vi "WriteSF.vi"(4 "error in":errorcluster, 5 "packet":u8[](array[numeric]), 6 "Enablle write":bool, 7 "connection ID":refnum<k5>) -> (0 "error out":errorcluster, 1 "Bytes written to SF":dbl, 2 "Packet String":string, 3 "connection ID out":refnum<k5>)   [LabVIEW 2011]
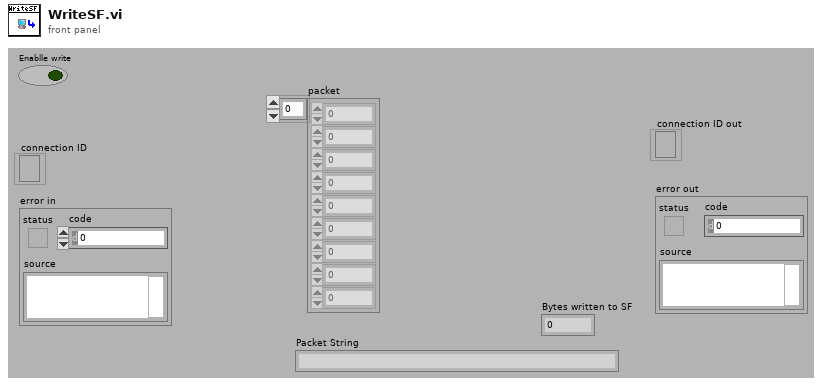
[diagram p1: front panel]
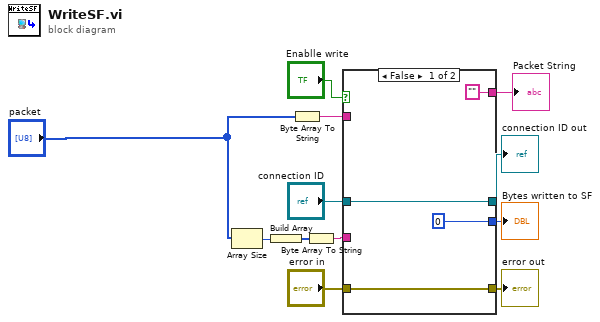
[diagram p0: block diagram]
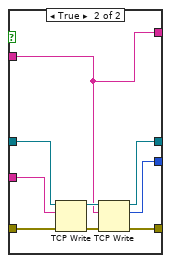
[diagram p2: hidden frame]
diagram:
  n1 = Array Size(array="packet") -> (size(s)=w2:i32)
  n2 = Build Array(w2) -> (w4:i32[])
  n3 = Byte Array To String(unsigned byte array="packet") -> (string=w6:string)
  n4 = Byte Array To String(unsigned byte array=w4) -> (string=w12:string)
  n5 = case shown="False" "Enablle write" {
    tunnel: "connection ID" -> [w16 w25]
    tunnel: "error in" -> [w15 w24]
    tunnel: [w16 w21] -> w9
    tunnel: [w15 w20] -> w10
    tunnel: [0 w19] -> w5
    tunnel: w6 -> [_ w17]
    tunnel: w12 -> [_ w18]
    tunnel: ["" ("string") w17] -> w3
    frame False {
    }
    frame True {
      n6 = TCP Write(connection ID=w25, data in=w18, error in (no error)=w24) -> (connection ID out=w22:refnum<k5>, error out=w23:errorcluster)  [unwired: 1 in, 1 out]
      n7 = TCP Write(connection ID=w22, data in=w17, error in (no error)=w23) -> (connection ID out=w21:refnum<k5>, bytes written=w19:i32, error out=w20:errorcluster)  [unwired: 1 in]
    }
  }
  "Bytes written to SF" <- w5
  "error out" <- w10
  "connection ID out" <- w9
  "Packet String" <- w3
